vi "Get Configuration Default.vi"(7 "Get Results Default? (F)":bool, 8 "error in (no error)":errorcluster, 11 "Measurement":refnum<class "MeasurementPluginService.lvclass">) -> (0 "error out":errorcluster, 3 "Control Default":variant)   [LabVIEW 2020, in "MeasurementLink Measurement Server.lvlib"]
uses:
  MeasurementLink Measurement Server.lvlib
  Classes/MeasurementPluginService/MeasurementPluginService.lvclass
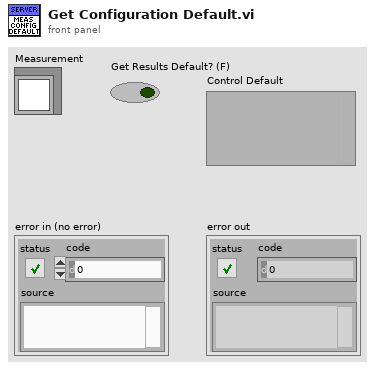
[diagram p1: front panel]
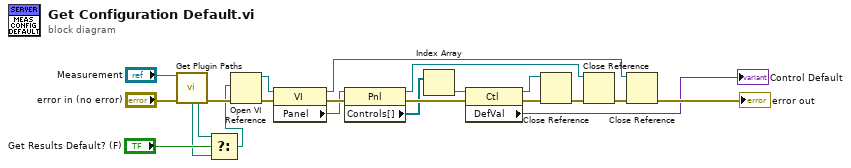
[diagram p0: block diagram]
diagram:
  n1 = call-dynamic "Get Plugin Paths.vi"("MeasurementService in"="Measurement", "error in (no error)"="error in (no error)") -> ("Measurement Configuration CTL Path"=w2:path, "Measurement Results CTL Path"=w3:path, "error out"=w4:errorcluster)  [unwired: 7 in, 4 out]
  n2 = Select(t=w3, s="Get Results Default? (F)", f=w2) -> (s? t:f=w1:path)
  n3 = Open VI Reference(vi path=w1, error in (no error)=w4) -> (vi reference=w10:refnum<vi>, error out=w19:errorcluster)  [unwired: 4 in]
  n4 = property class="VI"(reference=w10, error in=w19) -> (reference out=w15:refnum<vi>, error out=w18:errorcluster, "Panel"=w11:refnum<vi>)
  n5 = property class="Pnl"(reference=w11, error in=w18) -> (reference out=w14:refnum<vi>, error out=w20:errorcluster, "Controls[]"=w12:refnum<vi>[])
  n6 = Index Array(array=w12) -> (element=w21:refnum<vi>)  [unwired: 1 in]
  n7 = property class="Ctl"(reference=w21, error in=w20) -> (reference out=w13:refnum<vi>, error out=w22:errorcluster, "DefVal"=→"Control Default":variant)
  n8 = Close Reference(reference=w13, error in (no error)=w22) -> (error out=w17:errorcluster)
  n9 = Close Reference(reference=w14, error in (no error)=w17) -> (error out=w16:errorcluster)
  n10 = Close Reference(reference=w15, error in (no error)=w16) -> (error out=→"error out":errorcluster)
